vi "cunter.vi"(10 "input valid":bool, 11 "count to":u16) -> (2 "count":u16, 3 "reset (out)":bool)   [LabVIEW 2021]
uses:
  <vilib>/rvi/FXPMathLib/basic elements/FxpAddSub/XNode/nifxpmath_AddSub.xnode
  <vilib>/rvi/FXPMathLib/sim/FxpSim.dll
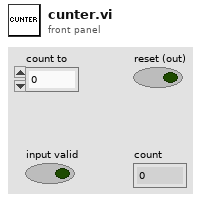
[diagram p1: front panel]
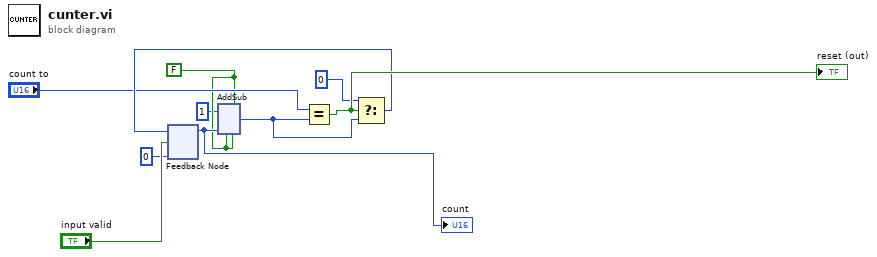
[diagram p0: block diagram]
diagram:
  w3 = FALSE ("use zero instead of x")
  n1 = feedback #1(u16 0 ("data index 3")) -> (w9:u16)
  "count" <- w9
  n2 = xnode "AddSub"("x"=u16 1, "y"=w9, "is sub?"=w3, "carry-in/inverted borrow-in"=w3, "use zero instead of x"=w3) -> ("s"=w5:u16)  [unwired: 1 out]
  n3 = Equal?(x="count to", y=w5) -> (x = y?=w8:bool)
  "reset (out)" <- w8
  n4 = Select(t=u16 0, s=w8, f=w5) -> (s? t:f=w7:u16)
  n5 = feedback-in #1(w7, "input valid") -> ()
